vi "RestoreSetupLVSource.vi"() -> ()   [LabVIEW 2021]
uses:
  <userlib>/_OpenG.lib/file/file.llb/Convert File Extension (Path)__ogtk.vi
  <userlib>/_OpenG.lib/lvzip/lvzip.llb/subVI/ZLIB Extract All Files To Dir (Path)__ogtk.vi
  <userlib>/_OpenG.lib/lvzip/fileutil.llb/subVIs/FILE Rename (Path)__ogtk.vi
  <vilib>/Wiresmith Technology/G CLI/CLI Class/CLI.lvclass
  <userlib>/_OpenG.lib/file/file.llb/openg_file.lvlib
  <vilib>/Utility/config.llb/NI_LVConfig.lvlib
panel:
  out "error out":errorcluster
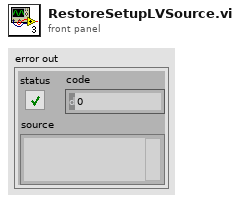
[diagram p1: front panel]
types:
  T1 = enum32{"Invalid", "Standard", "Closed", "Hidden", "Minimized", "Maximized"}
  T2 = typedef "NI_LVConfig.lvlib/Config Data RefNum.ctl" = refnum<k1>
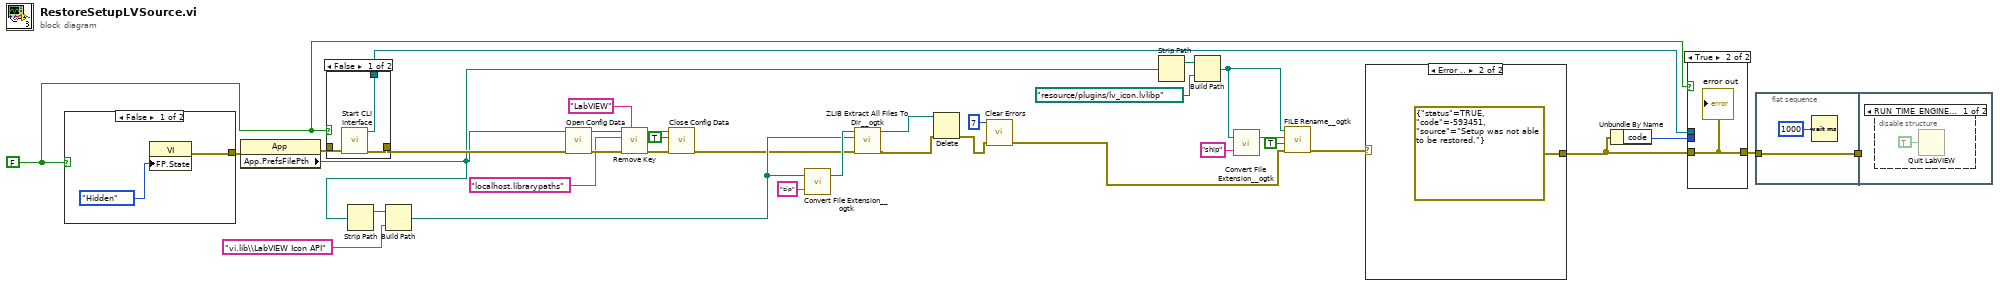
[diagram p0: block diagram]
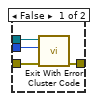
[diagram p3: hidden frame]
diagram:
  w11 = FALSE
  n1 = case shown="False" w11 {
    tunnel: [w36 _] -> w31
    frame False {
      n2 = property class="VI"("FP.State"=T1."Hidden" ("Front Panel Window:State")) -> (error out=w36:errorcluster)  [unwired: 2 in, 1 out]
    }
    frame True {
    }
  }
  n3 = property class="App"(error in=w31) -> (error out=w30:errorcluster, "App.PrefsFilePth"=w3:path)  [unwired: 1 in, 1 out]
  n4 = case shown="False" w11 {
    tunnel: [w40 _] -> w35
    tunnel: w30 -> [w39 w41]
    tunnel: [w38 w41] -> w18
    frame False {
      n5 = call <vilib>:"Start CLI Interface.vi"("error in (no error)"=w39) -> ("error out"=w38:errorcluster, "CLI out"=w40:refnum<class "CLI.lvclass">)  [unwired: 7 in, 2 out]
    }
    frame True {
    }
  }
  n6 = Strip Path(path=w3) -> (stripped path=w27:path)  [unwired: 1 out]
  n7 = Build Path(base path=w27, name or relative path="vi.lib\\LabVIEW Icon API" ("name")) -> (appended path=w25:path)
  n8 = call <vilib>:"Open Config Data.vi"("error in (no error)"=w18, "configuration file path"=w3) -> ("error out"=w22:errorcluster, "refnum"=w20:T2)  [unwired: 7 in, 1 out]
  n9 = call <vilib>:"Remove Key.vi"("section"="LabVIEW", "error in (no error)"=w22, "key"="localhost.librarypaths", "refnum"=w20) -> ("error out"=w21:errorcluster, "refnum out"=w19:T2)  [unwired: 5 in, 1 out]
  n10 = call <vilib>:"Close Config Data.vi"("error in (no error)"=w21, "write file if changed (T)"=TRUE, "refnum"=w19) -> ("error out"=w17:errorcluster)  [unwired: 7 in, 1 out]
  n11 = call-poly <userlib>:"Convert File Extension__ogtk.vi"("new ending (none)"="zip", "file name"=w25) -> ("new filename"=w26:path)  [unwired: 1 out]
  n12 = call-poly <userlib>:"ZLIB Extract All Files To Dir__ogtk.vi"("error in (no error)"=w17, "destination directory (archive name without ending)"=w25, "archive name (file dialog)"=w26) -> ("error out"=w24:errorcluster, "archive name out"=w23:path)  [unwired: 6 in, 1 out]
  n13 = Delete(path (use dialog)=w23, error in=w24) -> (error out=w13:errorcluster)  [unwired: 3 in, 2 out]
  n14 = call <vilib>:"Clear Errors.vi"("error in (no error)"=w13, "specific error code to clear (0: all)"=7) -> ("error out"=w4:errorcluster)  [unwired: 4 in, 1 out]
  n15 = Strip Path(path=w3) -> (stripped path=w10:path)  [unwired: 1 out]
  n16 = Build Path(base path=w10, name or relative path=path "resource/plugins/lv_icon.lvlibp") -> (appended path=w5:path)
  n17 = call-poly <userlib>:"Convert File Extension__ogtk.vi"("new ending (none)"="ship", "file name"=w5) -> ("new filename"=w6:path)  [unwired: 1 out]
  n18 = call-poly <userlib>:"FILE Rename__ogtk.vi"("error in (no error)"=w4, "overwrite (F)"=TRUE, "source path"=w6, "target path"=w5) -> ("error out"=w2:errorcluster)  [unwired: 6 in, 1 out]
  n19 = case shown="Error .." w2 {
    selector: w2 -> [w42 _]
    tunnel: [w42 errorcluster {"status"=TRUE, "code"=-593451, "source"="Setup was not able to be restored."} ("error out")] -> w1
    frame No Error {
    }
    frame Error {
    }
  }
  n20 = Unbundle By Name(w1) -> ("code"=w32:i32)
  n21 = case shown="True" w11 {
    tunnel: w35 -> [w47 _]
    tunnel: [w46 w48] -> w33
    tunnel: w32 -> [w45 _]
    tunnel: w1 -> [w44 w48]
    frame False {
      n22 = call <vilib>:"Exit With Error Cluster Code.vi"("error in (no error)"=w44, "No Error Code (0)"=w45, "CLI in"=w47) -> ("error out"=w46:errorcluster)  [unwired: 8 in]
    }
    frame True {
      "error out" <- w48
    }
  }
  n23 = flat-sequence {
    tunnel: w33 -> [w50]
    tunnel: [w50] -> w34
    tunnel: w34 -> [_]
    frame #0 {
      n24 = Wait (ms)(milliseconds to wait=u32 1000) -> ()  [unwired: 1 out]
    }
    frame #1 {
      n25 = disable-structure shown="RUN_TIME_ENGINE==True" {
        frame condition #0 {
          n26 = Quit LabVIEW(quit? (T)=TRUE) -> ()
        }
        frame condition #1 (active) {
        }
      }
    }
  }
